vi "Assembler Launcher.vi"() -> ()   [LabVIEW 2015]
uses:
  Test Actors/RandomDataChart/RandomDataChart.lvclass
  Test Actors/NumericCounter/NumericCounter.lvclass
  Test Actors/MultiSubscriber/MultiSubscriber.lvclass
  Test Actors/ConcreteViewModel/ConcreteViewModel.lvclass
  Test Actors/ValueInputs/ValueInputs.lvclass
  Test Actors/AutoRegPanel/AutoRegPanel.lvclass
  Test Actors/ActorAutoRegPanel/ActorAutoRegPanel.lvclass
  Framework/IViewModel/IViewModel/IViewModel.lvclass
  Framework/IViewable/IViewable/View Position Enum.ctl
  Framework/IModel/IModel/IModel.lvclass
  Framework/Mediator/Mediator/Mediator.lvclass
  <vilib>/ActorFramework/Message Enqueuer/Message Priority.ctl
  Test Actors/ConcreteModel/ConcreteModel.lvclass
  Framework/IViewModel/IViewModel/IViewModel.lvclass/IViewModel.ctl
  Framework/IViewManager/IViewManager Messages/Launch Nested Views Msg/Launch Nested Views Msg.lvclass/Launch Nested Views Msg.ctl
  Framework/IViewManager/IViewManager/IViewManager.lvclass/IViewManager.ctl
  Framework/IViewable/IViewable Messages/Show View Msg/Show View Msg.lvclass/Show View Msg.ctl
  <vilib>/ActorFramework/Message Enqueuer/Message Enqueuer.lvclass/Message Enqueuer.ctl
  Framework/IViewManager/IViewManager Messages/Launch Nested Views Msg/Build Launch Nested Views Msg.vi
  Framework/IViewManager/IViewManager/Write Startup Launch Nested Views Msg.vi
  <vilib>/ActorFramework/Message Enqueuer/Enqueue.vi
  <vilib>/ActorFramework/Message Priority Queue/Priority Enqueue.vi
  Framework/IViewManager/IViewManager Messages/Launch Nested Views Msg/Launch Nested Views Msg.lvclass
  Framework/IViewable/IViewable Messages/Show View Msg/Show View Msg.lvclass
  <vilib>/ActorFramework/Actor/Actor.lvclass
  ViewManager Implementations/LeftListboxViewManager/LeftListboxViewManager.lvclass
  ViewManager Implementations/TabbedViewManager/TabbedViewManager.lvclass
  ViewManager Implementations/QuadViewManager/QuadViewManager.lvclass
  Framework/IViewable/IViewable/IViewable.lvclass
  <vilib>/ActorFramework/Message Enqueuer/Message Enqueuer.lvclass
panel:
  out "error out":errorcluster
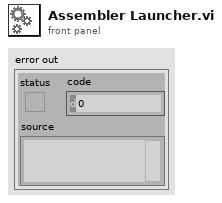
[diagram p1: front panel]
types:
  T1 = typedef "Actor Framework.lvlib/Message Enqueuer.lvclass/Message Priority.ctl" = enum16{"Low", "Normal", "High"}
  T2 = typedef "IViewable.lvlib/IViewable.lvclass/View Position Enum.ctl" = enum16{"Centered", "Maximized", "Minimized", "Custom", "Unchanged"}
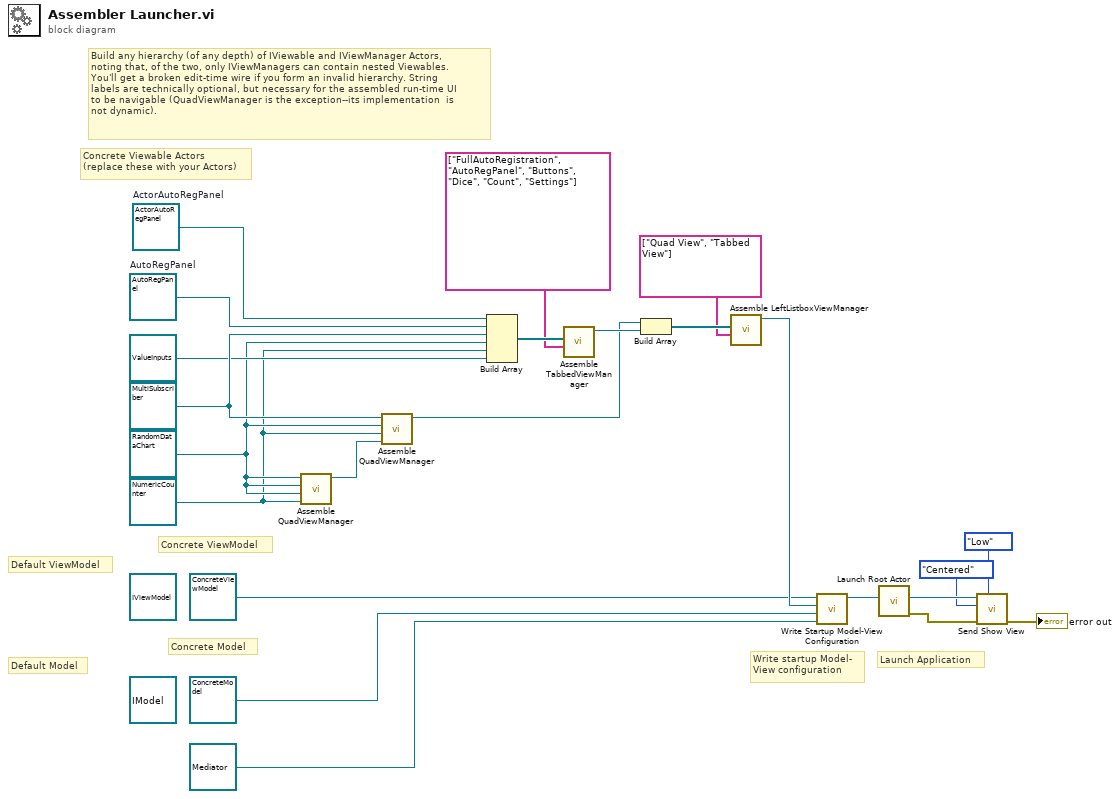
[diagram p0: block diagram]
diagram:
  (unwired) refnum<class "IModel.lvclass"> refnum ("IModel.lvlib:IModel.lvclass")
  (unwired) refnum<class "IViewModel.lvclass"> refnum ("IController.lvlib:IController.lvclass")
  w9 = refnum<class "ActorAutoRegPanel.lvclass"> refnum  # ActorAutoRegPanel
  w10 = refnum<class "AutoRegPanel.lvclass"> refnum  # AutoRegPanel
  w16 = refnum<class "MultiSubscriber.lvclass"> refnum ("TestActors.lvlib:ButtonPanel.lvclass")
  w13 = refnum<class "NumericCounter.lvclass"> refnum ("TestActors.lvlib:NumericCounter.lvclass")
  w14 = refnum<class "RandomDataChart.lvclass"> refnum ("TestActors.lvlib:RandomDataChart.lvclass")
  # "Concrete Model"
  # "Default Model"
  # "Default ViewModel"
  # "Concrete ViewModel"
  # "Concrete Viewable Actors\n(replace these with your Actors)"
  # "Launch Application"
  # "Write startup Model-\nView configuration"
  # "Build any hierarchy (of any depth) of IViewable and IViewManager Actors,\nnoting that, of the two, only IViewManagers can contain nested Viewables.\nYou'll get a broken edit-time wire if you form an invalid hierarchy. String\nlabels are technically optional, but necessary for the assembled run-time UI\nto be navigable (QuadViewManager is the exception--its implementation  is\nnot dynamic)."
  n1 = call "Assemble QuadViewManager.vi"("Bottom Right View"=w13, "Bottom Left View"=w14, "Top Right View"=w14, "Top Left View"=w14) -> ("QuadViewManager out"=w12:refnum<class "QuadViewManager.lvclass">)  [unwired: 7 in]
  n2 = call "Assemble QuadViewManager.vi"("Bottom Right View"=w12, "Bottom Left View"=w13, "Top Right View"=w14, "Top Left View"=w16) -> ("QuadViewManager out"=w11:refnum<class "QuadViewManager.lvclass">)  [unwired: 7 in]
  n3 = Build Array(w9, w10, w16, w14, w13, refnum<class "ValueInputs.lvclass"> refnum ("TestActors.lvlib:NumericInputs.lvclass")) -> (w22:refnum<class "IViewable.lvclass">[])
  n4 = call "Assemble TabbedViewManager.vi"("View Names"=string[] ["FullAutoRegistration", "AutoRegPanel", "Buttons", "Dice", "Count", "Settings"] ("View Labels"), "Views"=w22) -> ("TabbedViewManager Out"=w19:refnum<class "TabbedViewManager.lvclass">)  [unwired: 9 in]
  n5 = Build Array(w11, w19) -> (w21:refnum<class "IViewManager.lvclass">[])
  n6 = call "Assemble LeftListboxViewManager.vi"("View Names"=string[] ["Quad View", "Tabbed View"] ("View Labels"), "Views"=w21) -> ("LeftListboxViewManager Out"=w20:refnum<class "LeftListboxViewManager.lvclass">)  [unwired: 9 in]
  n7 = call "Write Startup Model-View Configuration.vi"("Mediator"=refnum<class "Mediator.lvclass"> refnum ("Mediator.lvlib:Mediator.lvclass"), "Model"=refnum<class "ConcreteModel.lvclass"> refnum ("TopLevelApplication.lvlib:ConcreteModel.lvclass"), "Startup View Configuration"=w20, "IViewModel In"=refnum<class "ConcreteViewModel.lvclass"> refnum ("TopLevelApplication.lvlib:TopLevelApplication.lvclass")) -> ("IViewModel Out"=w23:refnum<class "ConcreteViewModel.lvclass">)  [unwired: 7 in]
  n8 = call <vilib>:"Launch Root Actor.vi"("Actor"=w23) -> ("error out"=w6:errorcluster, "Actor's Enqueuer"=w8:refnum<class "Message Enqueuer.lvclass">)  [unwired: 9 in]
  n9 = call "Send Show View.vi"("Message Priority (Normal)"=Message_Priority."Low", "error in (no error)"=w6, "Position"=View_Position_Enum."Centered", "Message Enqueuer"=w8) -> ("error out"=→"error out":errorcluster)  [unwired: 6 in, 1 out]
